vi "Read Languages.vi"(8 "error in (no error)":errorcluster, 11 "GObject in":refnum<class "GObject.lvclass">) -> (0 "error out":errorcluster, 2 "Languages":T1[](array[typedef]), 3 "GObject out":refnum<class "GObject.lvclass">)   [LabVIEW 2013, in "SET Project Data.lvlib" / "GObject.lvclass"]
uses:
  GObject.lvclass
  Types/ProjFile_Language Entry.ctl
  GObject.lvclass/GObject.ctl
  Resource Data Class/Resource Data.lvclass/Resource Data.ctl
  Resource Data Class/Resource Data.lvclass
  SET Project Data.lvlib
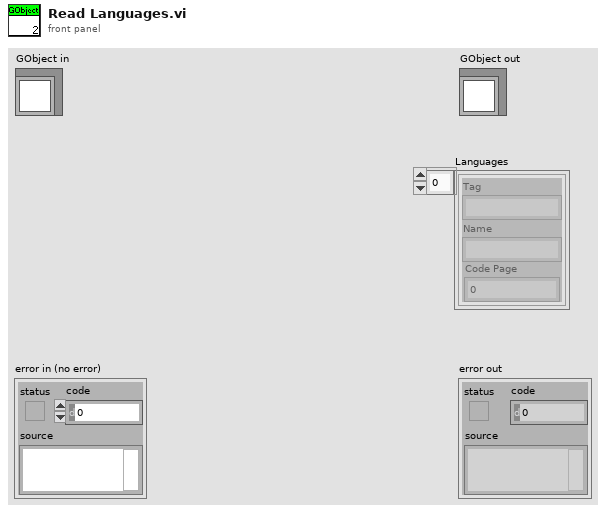
[diagram p1: front panel]
types:
  T1 = typedef "SET Project Data.lvlib/ProjFile_Language Entry.ctl" = cluster{"Tag":string, "Name":string, "Code Page":u16}
  T2 = typedef "SET Project Data.lvlib/ProjFile_Language Data.ctl" = cluster{"Tag":string, "Name":string, "Code Page":u16}
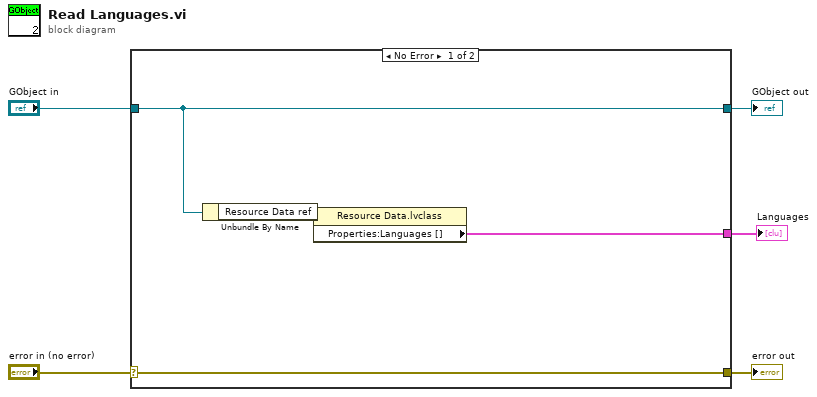
[diagram p0: block diagram]
diagram:
  n1 = case shown="No Error" "error in (no error)" {
    selector: "error in (no error)" -> [w9 w11]
    tunnel: [w9 w11] -> w4
    tunnel: [w8 w10] -> w2
    tunnel: "GObject in" -> [w8 w10]
    tunnel: [w6 _] -> w1
    frame No Error {
      n2 = Unbundle By Name(w8) -> ("Resource Data ref"=w7:refnum<data-value>)
      n3 = property class="Resource Data.lvclass"(reference=w7) -> ("Properties:Languages []"=w6:T2[])  [unwired: 1 in, 2 out]
    }
    frame Error {
    }
  }
  "error out" <- w4
  "GObject out" <- w2
  "Languages" <- w1
